vi "JagStatus.vi"(3 "Enable":bool) -> ()   [LabVIEW 2011]
uses:
  <vilib>/Rock Robotics/WPI/CAN/Jaguar/SubVIs/WPI_CANJaguar_StatusSelect.ctl
panel:
  in  "Motor Name":string(combo)
  out "Comm Fault":bool caption="Boolean"
  out "Gate Driver Fault":bool caption="Boolean"
  out "Bus Voltage Fault":bool caption="Boolean"
  out "Temperature Fault":bool caption="Boolean"
  out "Current Fault":bool caption="Boolean"
  out "Power Cycle":bool caption="Boolean"
  in  "Clear":bool
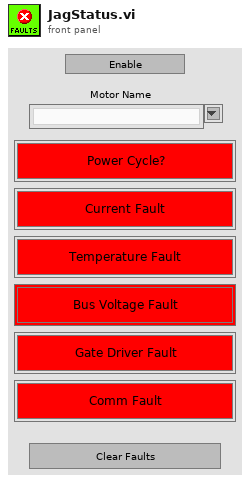
[diagram p1: front panel]
types:
  T1 = typedef "WPI_CANJaguar_StatusSelect.ctl" = enum16{"Output Percent VBus", "Output Voltage", "Bus Voltage", "Current", "Temperature", "Position", "Speed", "Limit Switches", "Faults", "Fault Counters", "Power Cycle"}
  T2 = typedef "WPI_MotorControlDeviceRef.ctl" = cluster{"DeviceStatus":errorcluster, "Type":enum16{"PWM", "CAN"}, "PWM":cluster{"Digital Module":T3, "PWM Channel":T4, "DeadBand":T5}, "CAN":cluster{"Device Number":u8, "Control Mode":T6, "Semaphore":T7, "Max Vout":dbl}, "Invert":bool, "TransformRef":T8, "InvTransformRef":T8}
  T3 = typedef "FPGA_TypedefDigitalModule.ctl" = enum16{"Digital Module 1", "Digital Module 2"}
  T4 = typedef "FPGA_DIOPWMChannel.ctl" = enum8{"PWM 1", "PWM 2", "PWM 3", "PWM 4", "PWM 5", "PWM 6", "PWM 7", "PWM 8", "PWM 9", "PWM 10", "Invalid"}
  T5 = typedef "WPI_PWMDeadband.ctl" = cluster{"Name":string, "maxPositivePwm":i32, "minPositivePwm":i32, "centerPwm":i32, "maxNegativePwm":i32, "minNegativePwm":i32, "angularRange":u16}
  T6 = typedef "WPI_CANJaguar_ControlMode.ctl" = enum8{"Percent VBus", "Current", "Speed", "Position", "Voltage"}
  T7 = typedef "Semaphore RefNum" = refnum<k1>
  T8 = typedef "WPI_PWMTransform_ConPane.ctl" = refnum<vi>
  T9 = typedef "WPI_CANJaguar_Status.ctl" = cluster{"Output Percent VBus":dbl, "Output Voltage":dbl, "Bus Voltage":dbl, "Current":dbl, "Temperature":dbl, "Position":dbl, "Speed":dbl, "Limits":cluster{"Forward Limit":bool, "Reverse Limit":bool, "Forward Soft Limit":bool, "Reverse Soft Limit":bool, "Sticky Forward Limit":bool, "Sticky Reverse Limit":bool, "Sticky Forward Soft Limit":bool, "Sticky Reverse Soft Limit":bool}, "Faults":cluster{"Current Fault":bool, "Temperature Fault":bool, "Bus Voltage Fault":bool, "Gate Driver Fault":bool, "Comm Fault":bool}, "Fault Counters":cluster{"Current Faults":u8, "Temperature Faults":u8, "Bus Voltage Faults":u8, "Gate Driver Faults":u8, "Comm Faults":u8, "CAN Status":u8, "CAN RX Errors":u8, "CAN TX Errors":u8}, "Power Cycle":bool}
  T10 = cluster{"Current Fault":bool, "Temperature Fault":bool, "Bus Voltage Fault":bool, "Gate Driver Fault":bool, "Comm Fault":bool}
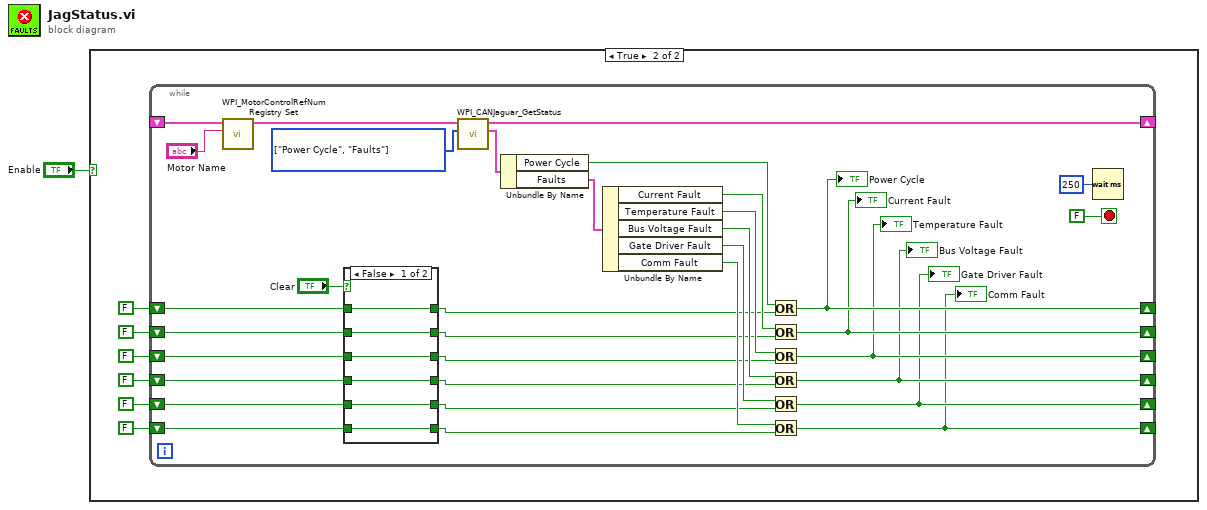
[diagram p0: block diagram]
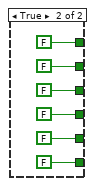
[diagram p3: hidden frame]
diagram:
  n1 = case shown="True" "Enable" {
    frame False {
    }
    frame True {
      n2 = while {
        shift-right: [w41] -> _
        shift-left: _ -> [w29]
        shift-right: [w15] -> _
        shift-left: FALSE -> [w26]
        shift-right: [w14] -> _
        shift-left: FALSE -> [w25]
        shift-right: [w13] -> _
        shift-left: FALSE -> [w24]
        shift-right: [w12] -> _
        shift-left: FALSE -> [w23]
        shift-right: [w11] -> _
        shift-left: FALSE -> [w22]
        shift-right: [w10] -> _
        shift-left: FALSE -> [w21]
        stop <- FALSE stop-if-true
        w40 = T1[] [enum."Power Cycle", enum."Faults"] items=["Output Percent VBus", "Output Voltage", "Bus Voltage", "Current", "Temperature", "Position", "Speed", "Limit Switches", "Faults", "Fault Counters", "Power Cycle"] ("Status Select")
        n3 = call <vilib>:"WPI_MotorControlRefNum Registry Set.vi"("refnum name"="Motor Name", "MotorControlDevRef"=w29) -> ("MotorControlDevRef"=w30:T2)  [unwired: 8 in, 1 out]
        n4 = case shown="False" "Clear" {
          tunnel: [w47 FALSE] -> w27
          tunnel: w26 -> [w47 _]
          tunnel: w25 -> [w46 _]
          tunnel: w24 -> [w45 _]
          tunnel: w23 -> [w44 _]
          tunnel: w22 -> [w43 _]
          tunnel: w21 -> [w42 _]
          tunnel: [w46 FALSE] -> w20
          tunnel: [w45 FALSE] -> w19
          tunnel: [w44 FALSE] -> w18
          tunnel: [w43 FALSE] -> w17
          tunnel: [w42 FALSE] -> w16
          frame False {
          }
          frame True {
          }
        }
        n5 = call <vilib>:"WPI_CANJaguar_GetStatus.vi"("Status Select"=w40, "CAN Jaguar Ref"=w30) -> ("Status"=w39:T9, "CAN Jaguar Ref Out"=w41:T2)  [unwired: 7 in, 1 out]
        n6 = Unbundle By Name(w39) -> ("Power Cycle"=w36:bool, "Faults"=w37:T10)
        n7 = Unbundle By Name(w37) -> ("Current Fault"=w35:bool, "Temperature Fault"=w34:bool, "Bus Voltage Fault"=w33:bool, "Gate Driver Fault"=w32:bool, "Comm Fault"=w31:bool)
        n8 = Or(x=w36, y=w27) -> (x .or. y?=w15:bool)
        "Power Cycle" <- w15
        n9 = Or(x=w35, y=w20) -> (x .or. y?=w14:bool)
        "Current Fault" <- w14
        n10 = Or(x=w34, y=w19) -> (x .or. y?=w13:bool)
        "Temperature Fault" <- w13
        n11 = Or(x=w33, y=w18) -> (x .or. y?=w12:bool)
        "Bus Voltage Fault" <- w12
        n12 = Or(x=w32, y=w17) -> (x .or. y?=w11:bool)
        "Gate Driver Fault" <- w11
        n13 = Or(x=w31, y=w16) -> (x .or. y?=w10:bool)
        "Comm Fault" <- w10
        n14 = Wait (ms)(milliseconds to wait=u32 250) -> ()  [unwired: 1 out]
      }
    }
  }
